vi "Virtual Motor.vi"(1 "dt":dbl=0.001, 2 "voltage":dbl[](array[knob]) scale=-5.0..5.0) -> (0 "theta":dbl[](array[knob]) scale=0.0..6.28)   [LabVIEW 2017]
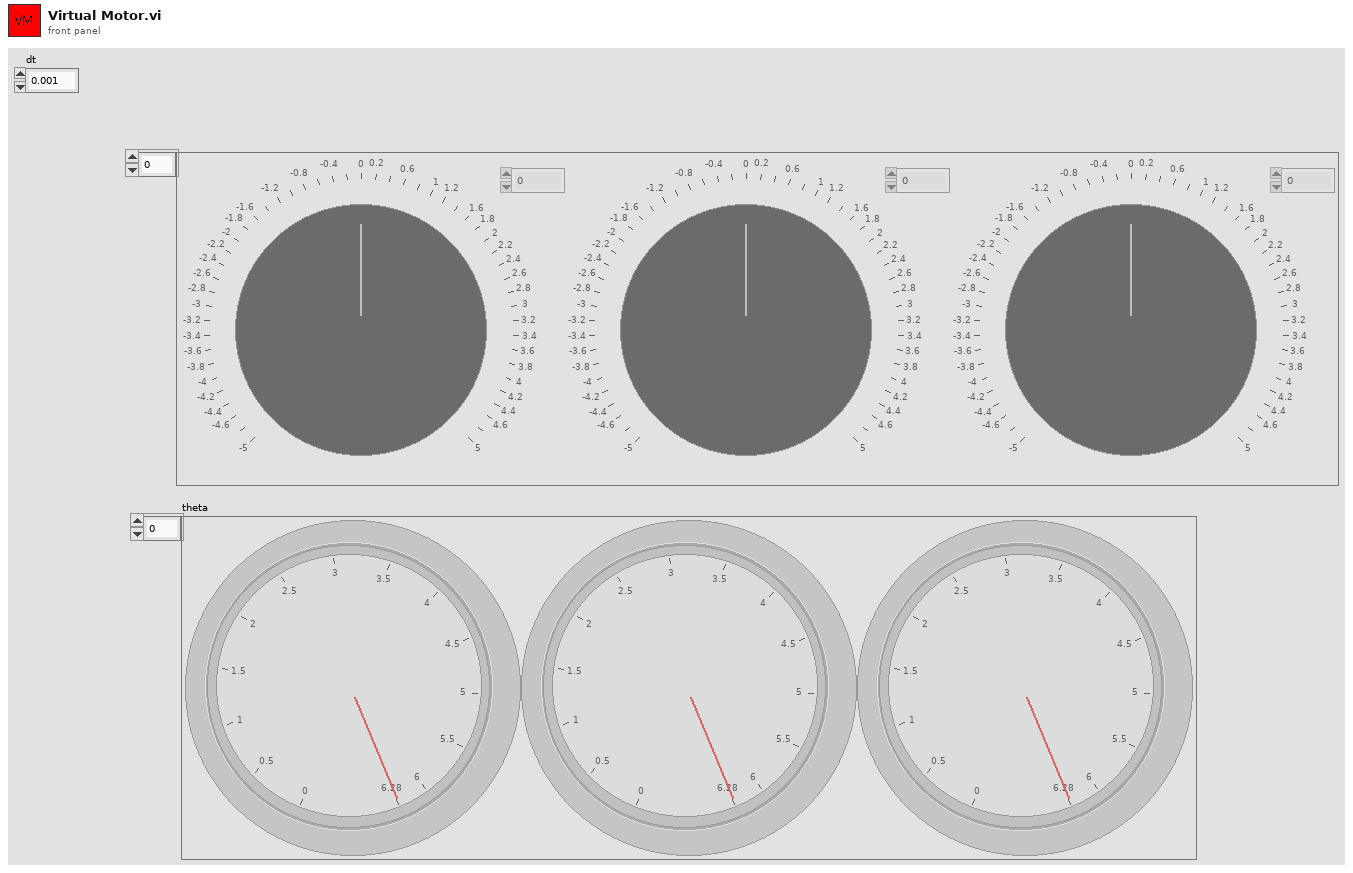
[diagram p1: front panel]
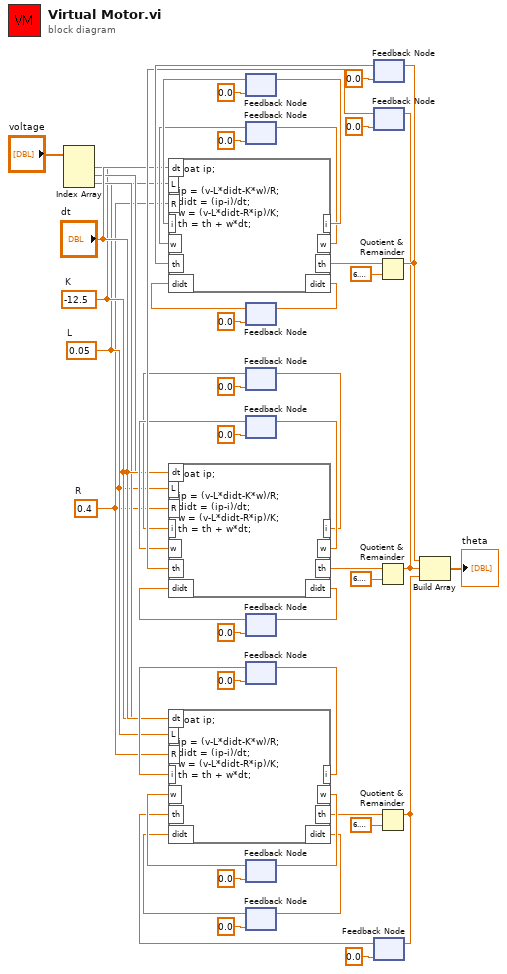
[diagram p0: block diagram]
diagram:
  w1 = 0.4  # R
  w2 = 0.05  # L
  w3 = -12.5  # K
  n1 = Index Array(array="voltage") -> (element #1=w11:dbl, element #2=w9:dbl, element #3=w8:dbl)  [unwired: 3 in]
  n2 = feedback #1(0.0 ("i")) -> (w50:dbl)
  n3 = feedback #2(0.0 ("w")) -> (w48:dbl)
  n4 = feedback #3(0.0 ("w")) -> (w39:dbl)
  n5 = feedback #4(0.0 ("i")) -> (w27:dbl)
  n6 = feedback #5(0.0 ("w")) -> (w29:dbl)
  n7 = feedback #6(0.0 ("w")) -> (w38:dbl)
  n8 = feedback #7(0.0 ("i")) -> (w24:dbl)
  n9 = feedback #8(0.0 ("w")) -> (w22:dbl)
  n10 = feedback #9(0.0 ("w")) -> (w13:dbl)
  n11 = feedback #10(0.0 ("w")) -> (w44:dbl)
  n12 = formula code="float ip;\n\nip = (v-L*didt-K*w)/R;\ndidt = (ip-i)/dt;\nw = (v-L*didt-R*ip)/K;\nth = th + w*dt;"("v"=w11, "K"=w3, "L"=w2, "R"=w1, "i"=w50, "w"=w48, "dt"="dt", "th"=w44, "didt"=w39) -> ("i"=w51:dbl, "w"=w49:dbl, "th"=w43:dbl, "didt"=w40:dbl)
  n13 = feedback-in #1(w51) -> ()
  n14 = feedback-in #2(w49) -> ()
  n15 = feedback-in #3(w40) -> ()
  n16 = feedback #11(0.0 ("w")) -> (w33:dbl)
  n17 = formula code="float ip;\n\nip = (v-L*didt-K*w)/R;\ndidt = (ip-i)/dt;\nw = (v-L*didt-R*ip)/K;\nth = th + w*dt;"("v"=w9, "K"=w3, "L"=w2, "R"=w1, "i"=w27, "w"=w29, "dt"="dt", "th"=w33, "didt"=w38) -> ("i"=w26:dbl, "w"=w28:dbl, "th"=w34:dbl, "didt"=w37:dbl)
  n18 = feedback-in #4(w26) -> ()
  n19 = feedback-in #5(w28) -> ()
  n20 = feedback-in #6(w37) -> ()
  n21 = feedback #12(0.0 ("w")) -> (w18:dbl)
  n22 = formula code="float ip;\n\nip = (v-L*didt-K*w)/R;\ndidt = (ip-i)/dt;\nw = (v-L*didt-R*ip)/K;\nth = th + w*dt;"("v"=w8, "K"=w3, "L"=w2, "R"=w1, "i"=w24, "w"=w22, "dt"="dt", "th"=w18, "didt"=w13) -> ("i"=w25:dbl, "w"=w23:dbl, "th"=w17:dbl, "didt"=w14:dbl)
  n23 = feedback-in #7(w25) -> ()
  n24 = feedback-in #8(w23) -> ()
  n25 = feedback-in #9(w14) -> ()
  n26 = Quotient & Remainder(x=w43, y=6.283185307179586) -> (x-y*floor(x/y)=w7:dbl)  [unwired: 1 out]
  n27 = feedback-in #10(w7) -> ()
  n28 = Quotient & Remainder(x=w34, y=6.283185307179586) -> (x-y*floor(x/y)=w5:dbl)  [unwired: 1 out]
  n29 = feedback-in #11(w5) -> ()
  n30 = Quotient & Remainder(x=w17, y=6.283185307179586) -> (x-y*floor(x/y)=w4:dbl)  [unwired: 1 out]
  n31 = feedback-in #12(w4) -> ()
  n32 = Build Array(w7, w5, w4) -> (→"theta":dbl[])
